vi "LM3Sxxxx_Watchdog_Config.vi"(8 "error in (no error)":errorcluster, 10 "Config Data":string[](array[string]), 11 "Interrupt Name":string) -> (0 "error out":errorcluster, 3 "Interrupt Configuration":string[](array[string]))   [LabVIEW 2011]
panel:
  in  "Lock registers":bool
  in  "help":bool
  in  "Reset timer":u32=1000
  in  "cancel":bool
  in  "ok":bool
  in  "Timer units":i32(ring)=1 items=["Milliseconds"=1, "Microseconds"=2, "Cycles"=0]
  # "The watchdog is not enabled in\ndebug mode."
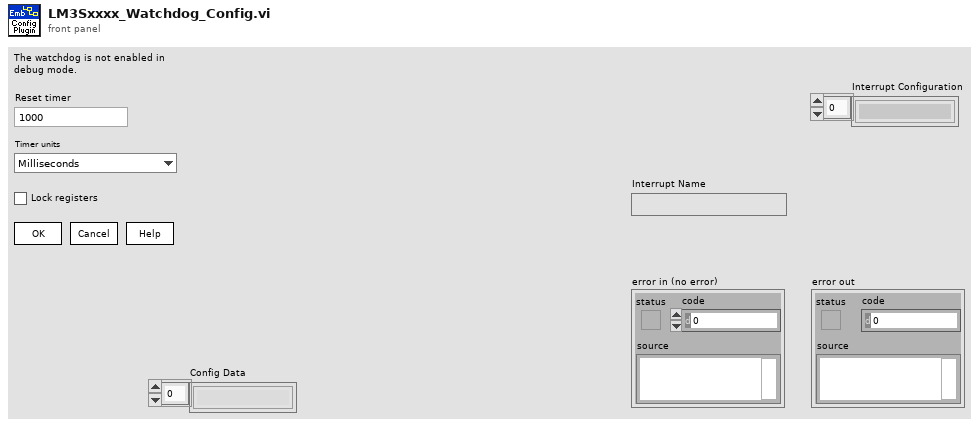
[diagram p1: front panel]
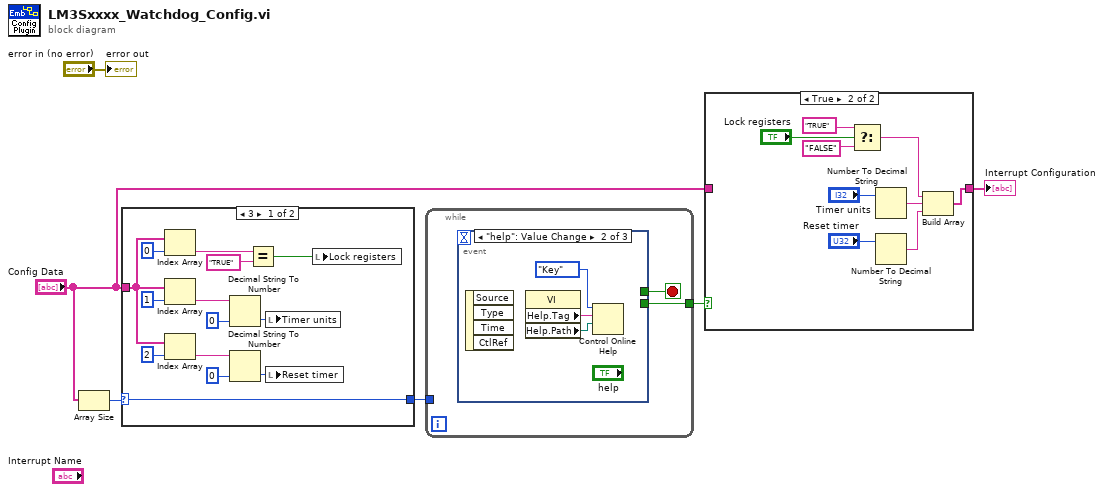
[diagram p0: block diagram]
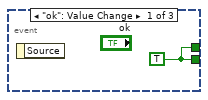
[diagram p4: hidden frame]
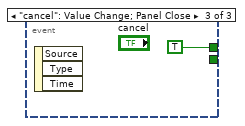
[diagram p5: hidden frame]
diagram:
  n1 = Array Size(array="Config Data") -> (size(s)=w5:i32)
  n2 = case shown="3" w5 {
    selector: w5 -> [w20 w21]
    tunnel: "Config Data" -> [w19 _]
    tunnel: [w20 w21] -> w4
    frame 3 {
      n3 = Index Array(array=w19, index=0) -> (element=w13:string)
      n4 = Index Array(array=w19, index=1) -> (element=w10:string)
      n5 = Index Array(array=w19, index=2) -> (element=w15:string)
      n6 = Decimal String To Number(string=w10, default (0L)=0) -> (number=w8:i32)  [unwired: 1 in, 1 out]
      n7 = Decimal String To Number(string=w15, default (0L)=u32 0 ("default (0 I32)")) -> (number=w14:u32)  [unwired: 1 in, 1 out]
      n8 = Equal?(x=w13, y="TRUE") -> (x = y?=w11:bool)
      n9 = local write "Timer units"(w8) -> ()
      n10 = local write "Reset timer"(w14) -> ()
      n11 = local write "Lock registers"(w11) -> ()
    }
    frame Default {
    }
  }
  n12 = while {
    tunnel: [w22] -> w3
    tunnel: w4 -> [_]
    stop <- w23 stop-if-true
    n13 = event shown="[1] \"help\": Value Change" {
      selector: _ -> [_ _ _]
      dyn-events: _ -> [_ _ _]
      timeout: _ -> [_ _ _]
      tunnel: [w24 _ TRUE] -> w23
      tunnel: [w24 _ _] -> w22
      event "ok": Value Change {
        w24 = TRUE
        n14 = event-data() -> ()  [unwired: 2 out]
      }
      event "help": Value Change {
        n15 = event-data() -> ()  [unwired: 5 out]
        n16 = property class="VI"() -> ("Help.Tag"=w25:string, "Help.Path"=w26:path)  [unwired: 2 in, 2 out]
        n17 = Control Online Help(2:w26, 3:w25, 4:enum16{"Contents", "Key", "Close"}."Key" ("Operation")) -> ()  [unwired: 1 in, 1 out]
      }
      event "cancel": Value Change; Panel Close {
        n18 = event-data() -> ()  [unwired: 4 out]
      }
    }
  }
  n19 = case shown="True" w3 {
    tunnel: "Config Data" -> [w29 _]
    tunnel: [w29 w32] -> w1
    frame False {
    }
    frame True {
      n20 = Select(t="TRUE", s="Lock registers", f="FALSE") -> (s? t:f=w35:string)
      n21 = Number To Decimal String(number="Timer units") -> (decimal integer string=w30:string)  [unwired: 1 in]
      n22 = Number To Decimal String(number="Reset timer") -> (decimal integer string=w33:string)  [unwired: 1 in]
      n23 = Build Array(w35, w30, w33) -> (w32:string[])
    }
  }
  "Interrupt Configuration" <- w1
  "error out" <- "error in (no error)"
